vi "Timer Status.vi"(8 "error in (no error)":errorcluster, 11 "Timer Demo App in":refnum<class "Timer Demo App.lvclass">) -> (0 "error out":errorcluster, 1 "Running":bool, 2 "Elapsed":dbl, 3 "Timer Demo App out":refnum<class "Timer Demo App.lvclass">)   [LabVIEW 2020, in "Timer Demo.lvlib" / "Timer Demo App.lvclass"]
uses:
  Timer Demo App.lvclass
  Timer Demo App.lvclass/Timer Demo App.ctl
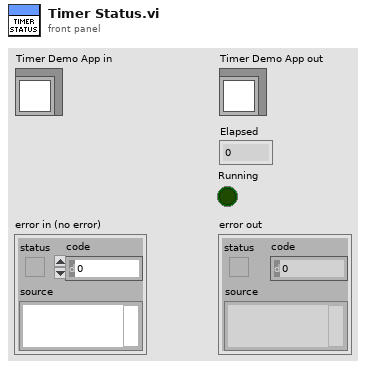
[diagram p1: front panel]
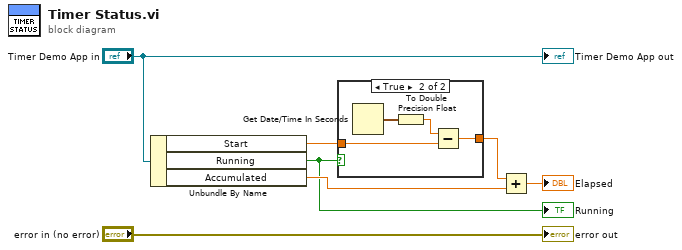
[diagram p0: block diagram]
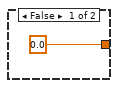
[diagram p2: hidden frame]
diagram:
  n1 = Unbundle By Name("Timer Demo App in") -> ("Start"=w2:dbl, "Running"=w3:bool, "Accumulated"=w5:dbl)
  "Running" <- w3
  n2 = case shown="True" w3 {
    tunnel: w2 -> [_ w11]
    tunnel: [0.0 w9] -> w1
    frame False {
    }
    frame True {
      n3 = Get Date/Time In Seconds() -> (seconds since 1Jan1904=w12:timestamp)
      n4 = To Double Precision Float(number=w12) -> (double precision float=w10:dbl)
      n5 = Subtract(x=w10, y=w11) -> (x-y=w9:dbl)
    }
  }
  n6 = Add(x=w1, y=w5) -> (x+y=→"Elapsed":dbl)
  "error out" <- "error in (no error)"
  "Timer Demo App out" <- "Timer Demo App in"
